vi "子VI-深度学习自动检测.vi"() -> ()   [LabVIEW 2018]
panel:
  out "预测图片原始路径":path
  in  "stop":bool caption="停止"
  in  "选项卡控件":enum32{"选项卡 1", "选项卡 2"}(tab)
  out "原图":T1(plugin-control)
  out "预测输出":T1(plugin-control)
  out "standard output":string caption="模型计算输出"
  out "穿透图原始路径":path
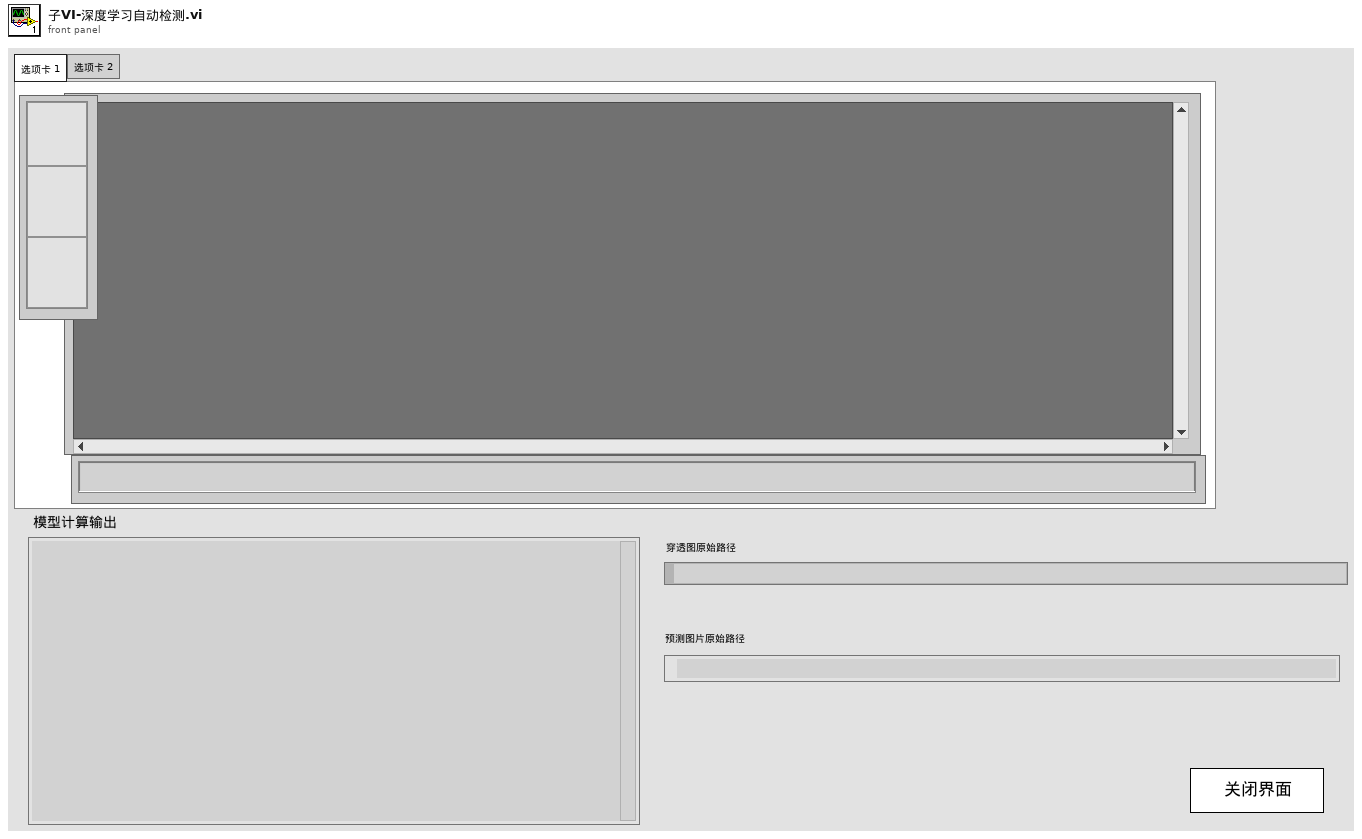
[diagram p1: front panel]
types:
  T1 = typedef "IMAQ Image.ctl" = refnum<image>
  T2 = typedef "Image Type" = u32
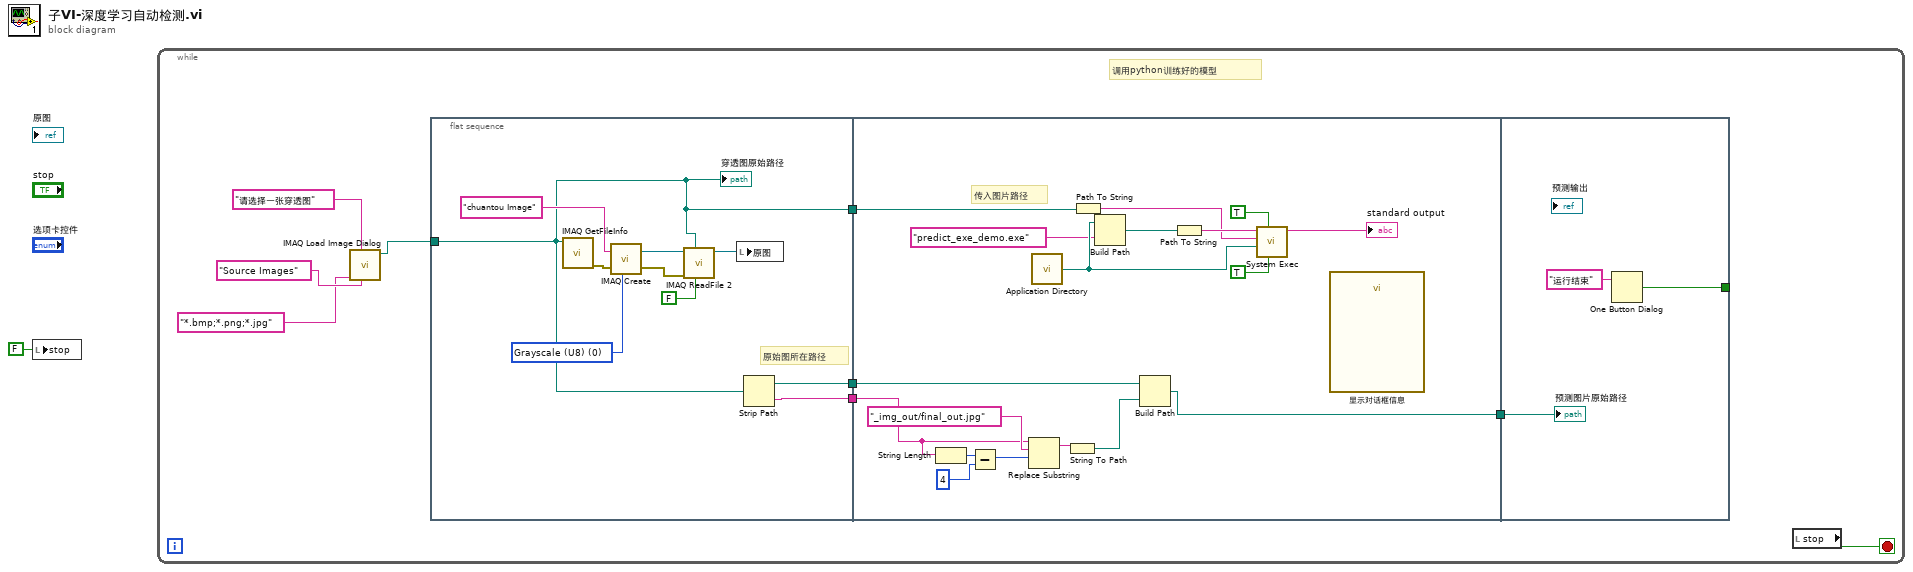
[diagram p0: block diagram]
diagram:
  n1 = local write "stop"(FALSE ("stop")) -> ()
  n2 = while {
    stop <- w5 stop-if-true
    # "调用python训练好的模型"
    n3 = call "IMAQ Load Image Dialog"("Pattern Label"="Source Images", "Prompt"="请选择一张穿透图" ("prompt"), "Pattern"="*.bmp;*.png;*.jpg") -> ("Path"=w6:path)  [unwired: 6 in, 2 out]
    n4 = flat-sequence {
      tunnel: w6 -> [w13]
      tunnel: [w13] -> w10
      tunnel: [w12] -> w4
      tunnel: [w11] -> w3
      tunnel: w10 -> [w32]
      tunnel: w4 -> [w29]
      tunnel: w3 -> [w22]
      tunnel: [w21] -> w2
      tunnel: [w40] -> _
      tunnel: w2 -> [w39]
      frame #0 {
        w15 = T2 0 items=["Grayscale (U8)", "Grayscale (I16)", "Grayscale (SGL)", "Complex (CSG)", "RGB (U32)", "HSL (U32)", "RGB (U64)", "Grayscale (U16)"] ("Image Type")
        # "原始图所在路径"
        n5 = call "IMAQ GetFileInfo"("File Path"=w13) -> ("error out"=w18:errorcluster)  [unwired: 4 in, 6 out]
        n6 = call "IMAQ Create"("Image Name"="chuantou Image", "Image Type"=w15, "error in (no error)"=w18) -> ("New Image"=w19:T1, "error out"=w20:errorcluster)  [unwired: 2 in]
        n7 = call "IMAQ ReadFile 2"("Use File Path Image Type"=FALSE, "File Path"=w13, "error in (no error)"=w20, "Image"=w19) -> ("Image Out"=w17:T1)  [unwired: 3 in, 4 out]
        n8 = local write "原图"(w17) -> ()
        n9 = Strip Path(path=w13) -> (stripped path=w12:path, name=w11:string)
        "穿透图原始路径" <- w13
      }
      frame #1 {
        # "传入图片路径"
        n10 = String Length(string=w22) -> (length=w27:i32)
        n11 = Subtract(x=w27, y=4) -> (x-y=w26:i32)
        n12 = Replace Substring(3:w26, 4:"_img_out/final_out.jpg" ("字符串"), 5:w22) -> (1:w28:string)  [unwired: 1 in, 1 out]
        n13 = call <vilib>:"Application Directory.vi"() -> ("Application Directory"=w36:path)
        n14 = String To Path(string=w28) -> (path=w23:path)
        n15 = Path To String(path=w32) -> (string=w31:string)
        n16 = Build Path(base path=w36, name or relative path="predict_exe_demo.exe" ("名称或相对路径")) -> (appended path=w37:path)
        n17 = Build Path(base path=w29, name or relative path=w23) -> (appended path=w21:path)
        n18 = Path To String(path=w37) -> (string=w38:string)
        n19 = call <vilib>:"System Exec.vi"("run minimized? (F)"=TRUE, "wait until completion? (T)"=TRUE, "working directory"=w36, "standard input"=w31, "command line"=w38) -> ("standard output"=→"standard output":string)  [unwired: 3 in, 3 out]
        n20 = call "显示对话框信息"() -> ()  [unwired: 10 in, 2 out]
      }
      frame #2 {
        n21 = One Button Dialog(message="运行结束" ("消息")) -> (true=w40:bool)  [unwired: 1 in]
        "预测图片原始路径" <- w39
      }
    }
    n22 = local read "stop"() -> (w5:bool)
  }
